vi "add RP100 scan T and voltage.vi"(11 "字符串 2":string) -> (1 "ok or cancel":bool, 3 "连接的字符串 2":string)   [LabVIEW 2019]
panel:
  in  "interval":dbl
  in  "电压 (V) 2":dbl
  in  "cancel 2":bool
  in  "ok 2":bool
  in  "电压 (V)":dbl
  in  "slew (V/sec）":dbl=1.0
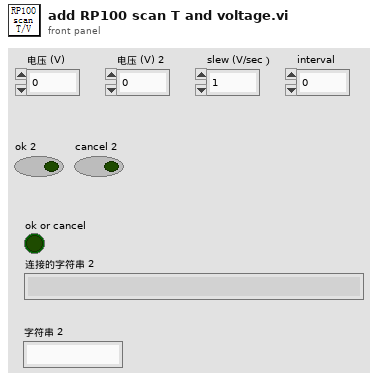
[diagram p1: front panel]
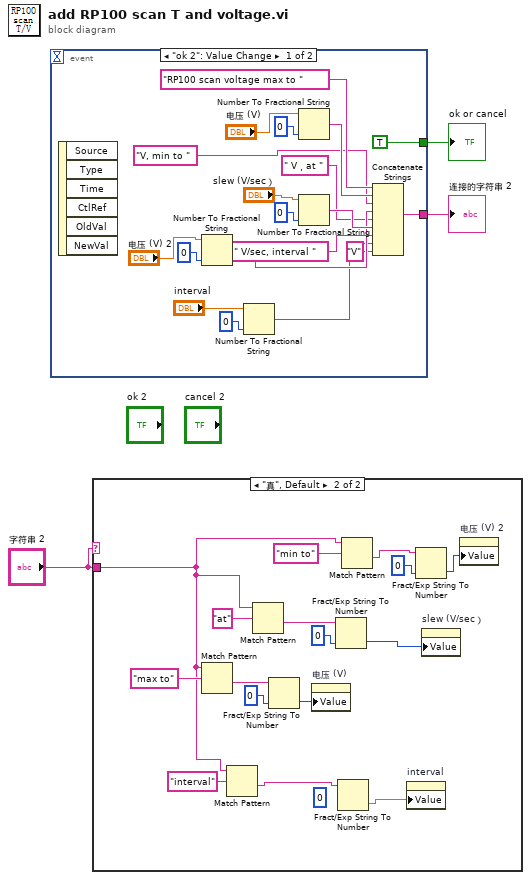
[diagram p0: block diagram]
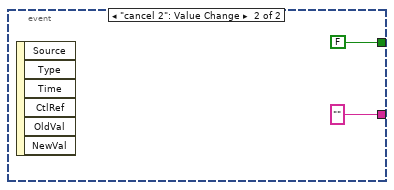
[diagram p3: hidden frame]
diagram:
  n1 = event shown="[0] \"ok 2\": Value Change" {
    selector: _ -> [_ _]
    dyn-events: _ -> [_ _]
    timeout: _ -> [_ _]
    tunnel: [TRUE FALSE] -> w2
    tunnel: [w16 "" ("分隔符")] -> w3
    event "ok 2": Value Change {
      n2 = event-data() -> ()  [unwired: 1 in, 6 out]
      n3 = Number To Fractional String(number="电压 (V) 2", precision (6)=i16 0 ("精度(6)")) -> (F-format string=w10:string)  [unwired: 2 in]
      n4 = Number To Fractional String(number="interval", precision (6)=i16 0 ("精度(6)")) -> (F-format string=w6:string)  [unwired: 2 in]
      n5 = Number To Fractional String(number="电压 (V)", precision (6)=i16 0 ("精度(6)")) -> (F-format string=w13:string)  [unwired: 2 in]
      n6 = Number To Fractional String(number="slew (V/sec）", precision (6)=i16 0 ("精度(6)")) -> (F-format string=w18:string)  [unwired: 2 in]
      n7 = Concatenate Strings("RP100 scan voltage max to " ("字符串"), w13, "V, min to " ("string"), w10, " V，at " ("字符串"), w18, " V/sec, interval " ("字符串"), w6, "V" ("string")) -> (w16:string)
    }
    event "cancel 2": Value Change {
      n8 = event-data() -> ()  [unwired: 1 in, 6 out]
    }
  }
  "ok or cancel" <- w2
  "连接的字符串 2" <- w3
  n9 = case shown="\"真\", Default" "字符串 2" {
    tunnel: "字符串 2" -> [_ w28]
    frame "" {
    }
    frame "真", Default {
      (unwired) 0
      n10 = Match Pattern(string=w28, regular expression="max to" ("正则表达式")) -> (after substring=w38:string)  [unwired: 1 in, 3 out]
      n11 = Match Pattern(string=w28, regular expression="interval") -> (after substring=w26:string)  [unwired: 1 in, 3 out]
      n12 = Match Pattern(string=w28, regular expression="at" ("正则表达式")) -> (after substring=w35:string)  [unwired: 1 in, 3 out]
      n13 = Fract/Exp String To Number(string=w38, default (0 dbl)=0) -> (number=w34:i32)  [unwired: 2 in, 1 out]
      n14 = property on="电压 (V)" class="DigNum (strict)"("Value"=w34) -> ()  [unwired: 2 in, 2 out]
      n15 = Fract/Exp String To Number(string=w35, default (0 dbl)=0) -> (number=w33:i32)  [unwired: 2 in, 1 out]
      n16 = Fract/Exp String To Number(string=w26) -> (number=w25:dbl)  [unwired: 3 in, 1 out]
      n17 = Match Pattern(string=w28, regular expression="min to" ("正则表达式")) -> (after substring=w30:string)  [unwired: 1 in, 3 out]
      n18 = property on="interval" class="DigNum (strict)"("Value"=w25) -> ()  [unwired: 2 in, 2 out]
      n19 = Fract/Exp String To Number(string=w30, default (0 dbl)=0) -> (number=w29:i32)  [unwired: 2 in, 1 out]
      n20 = property on="slew (V/sec）" class="DigNum (strict)"("Value"=w33) -> ()  [unwired: 2 in, 2 out]
      n21 = property on="电压 (V) 2" class="DigNum (strict)"("Value"=w29) -> ()  [unwired: 2 in, 2 out]
    }
  }
